vi "Drive Process.vi"   [LabVIEW 2013]
uses:
  Drive Global.vi
types:
  T1 = cluster{"X Axis":dbl, "Y Axis":dbl, "Slow Drive":bool, "Show Off Spin":bool, "Hands Off":bool, "Right Gear Distance":dbl, "Left Gear Distance ":dbl, "Right Gear RPM":dbl, "Left Gear RPM":dbl}
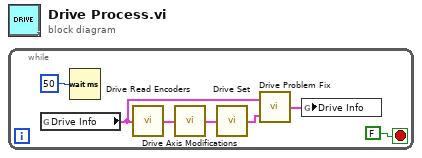
[diagram p0: block diagram]
diagram:
  n1 = while {
    stop <- FALSE stop-if-true
    n2 = global read "Drive Global.vi" "Drive Info"() -> (w2:T1)
    n3 = Wait (ms)(milliseconds to wait=u32 50) -> ()  [unwired: 1 out]
    n4 = call "Drive Read Encoders.vi"("Drive Info"=w2) -> ("Drive Out"=w4:T1)
    n5 = call "Drive Axis Modifications.vi"("Drive Info In"=w4) -> ("Drive Info Out"=w5:T1)
    n6 = call "Drive Set.vi"("Drive Info In"=w5) -> ("Drive Info Out"=w3:T1)
    n7 = call "Drive Problem Fix.vi"("Drive Info Modified"=w3, "Drive Info Original"=w2) -> ("Drive Info Fixed"=w1:T1)
    n8 = global write "Drive Global.vi" "Drive Info"(w1) -> ()
  }
